vi "Read MongoDB.Collection.vi"(8 "error in (no error)":errorcluster, 11 "MongoDB.Collection in":refnum<class "MongoDB.Collection.lvclass">) -> (0 "error out":errorcluster, 3 "MongoDB.Collection out":refnum<class "MongoDB.Collection.lvclass">)   [LabVIEW 2014, in "MongoDB.Collection.lvclass"]
uses:
  MongoDB.Collection.lvclass
  C:/Users/Richard/Documents/GitHub/mongo-labview-driver/CSharp/bin/MongoDB.Driver.Legacy.dll
  CSharp/bin/MongoDB.Driver.Legacy.dll
  MongoDB.Collection.lvclass/MongoDB.Collection.ctl
panel:
  out "MongoDB.Collection":refnum<k24>
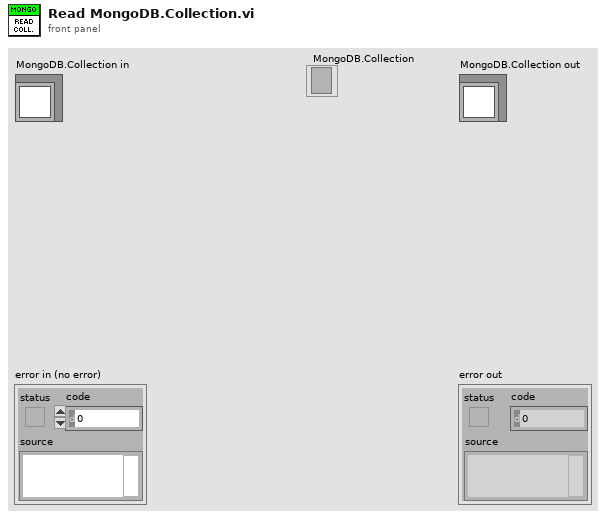
[diagram p1: front panel]
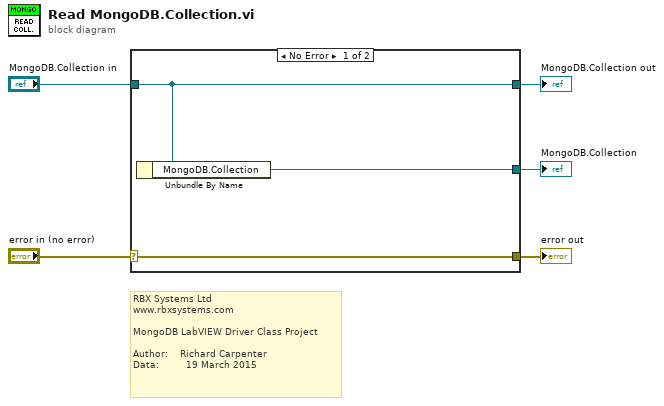
[diagram p0: block diagram]
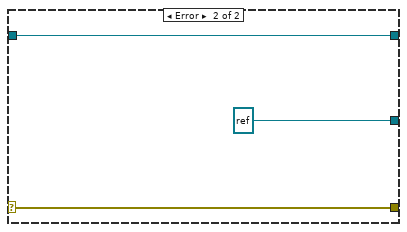
[diagram p2: hidden frame]
diagram:
  # "RBX Systems Ltd\nwww.rbxsystems.com\n\nMongoDB LabVIEW Driver Class Project\n\nAuthor:    Richard Carpenter\nData:         19 March 2015"
  n1 = case shown="No Error" "error in (no error)" {
    selector: "error in (no error)" -> [w8 w10]
    tunnel: [w8 w10] -> w4
    tunnel: [w7 w11] -> w2
    tunnel: "MongoDB.Collection in" -> [w7 w11]
    tunnel: [w6 refnum<k24> refnum ("MongoDB.Collection")] -> w1
    frame No Error {
      n2 = Unbundle By Name(w7) -> ("MongoDB.Collection"=w6:refnum<k24>)
    }
    frame Error {
    }
  }
  "error out" <- w4
  "MongoDB.Collection out" <- w2
  "MongoDB.Collection" <- w1
